vi "camera.vi"() -> (0 "color":string, 1 "result":bool, 2 "middle":T3(plugin-control))   [LabVIEW 2017]
panel:
  in  "range of detect screen":dbl=7.0
  in  "value of screen mid":dbl=160.0
  in  "distance between pole lines":sgl=2.0
  in  "Rectangle":T1={"Left"=150, "Top"=20, "Right"=170, "Bottom"=120, "Rotation"=0.0} {"Rotation" min=-90.0 max=90.0 step=1.0 format="%.2f"; "Left" scale=0.0..1024.0; "Right" scale=0.0..1024.0}
  out "inRange":bool
  out "not same":bool
  out "line_leftX":sgl
  out "line_rightX":sgl
  out "line_left":T2 {"Point2 (Real-World)"."Y" format="%.2f"; "Point2 (Real-World)"."X" format="%.2f"; "Point1 (Real-World)"."Y" format="%.2f"; "Point1 (Real-World)"."X" format="%.2f"; "Point2 (Pixels)"."Y" format="%.2f"; "Point2 (Pixels)"."X" format="%.2f"; "Point1 (Pixels)"."Y" format="%.2f"; "Point1 (Pixels)"."X" format="%.2f"}
  out "line_right":T2 {"Point2 (Real-World)"."Y" format="%.2f"; "Point2 (Real-World)"."X" format="%.2f"; "Point1 (Real-World)"."Y" format="%.2f"; "Point1 (Real-World)"."X" format="%.2f"; "Point2 (Pixels)"."Y" format="%.2f"; "Point2 (Pixels)"."X" format="%.2f"; "Point1 (Pixels)"."Y" format="%.2f"; "Point1 (Pixels)"."X" format="%.2f"}
  out "thresh":T3(plugin-control)
  in  "Stop (F)":bool
  out "Image Out":T3(plugin-control)
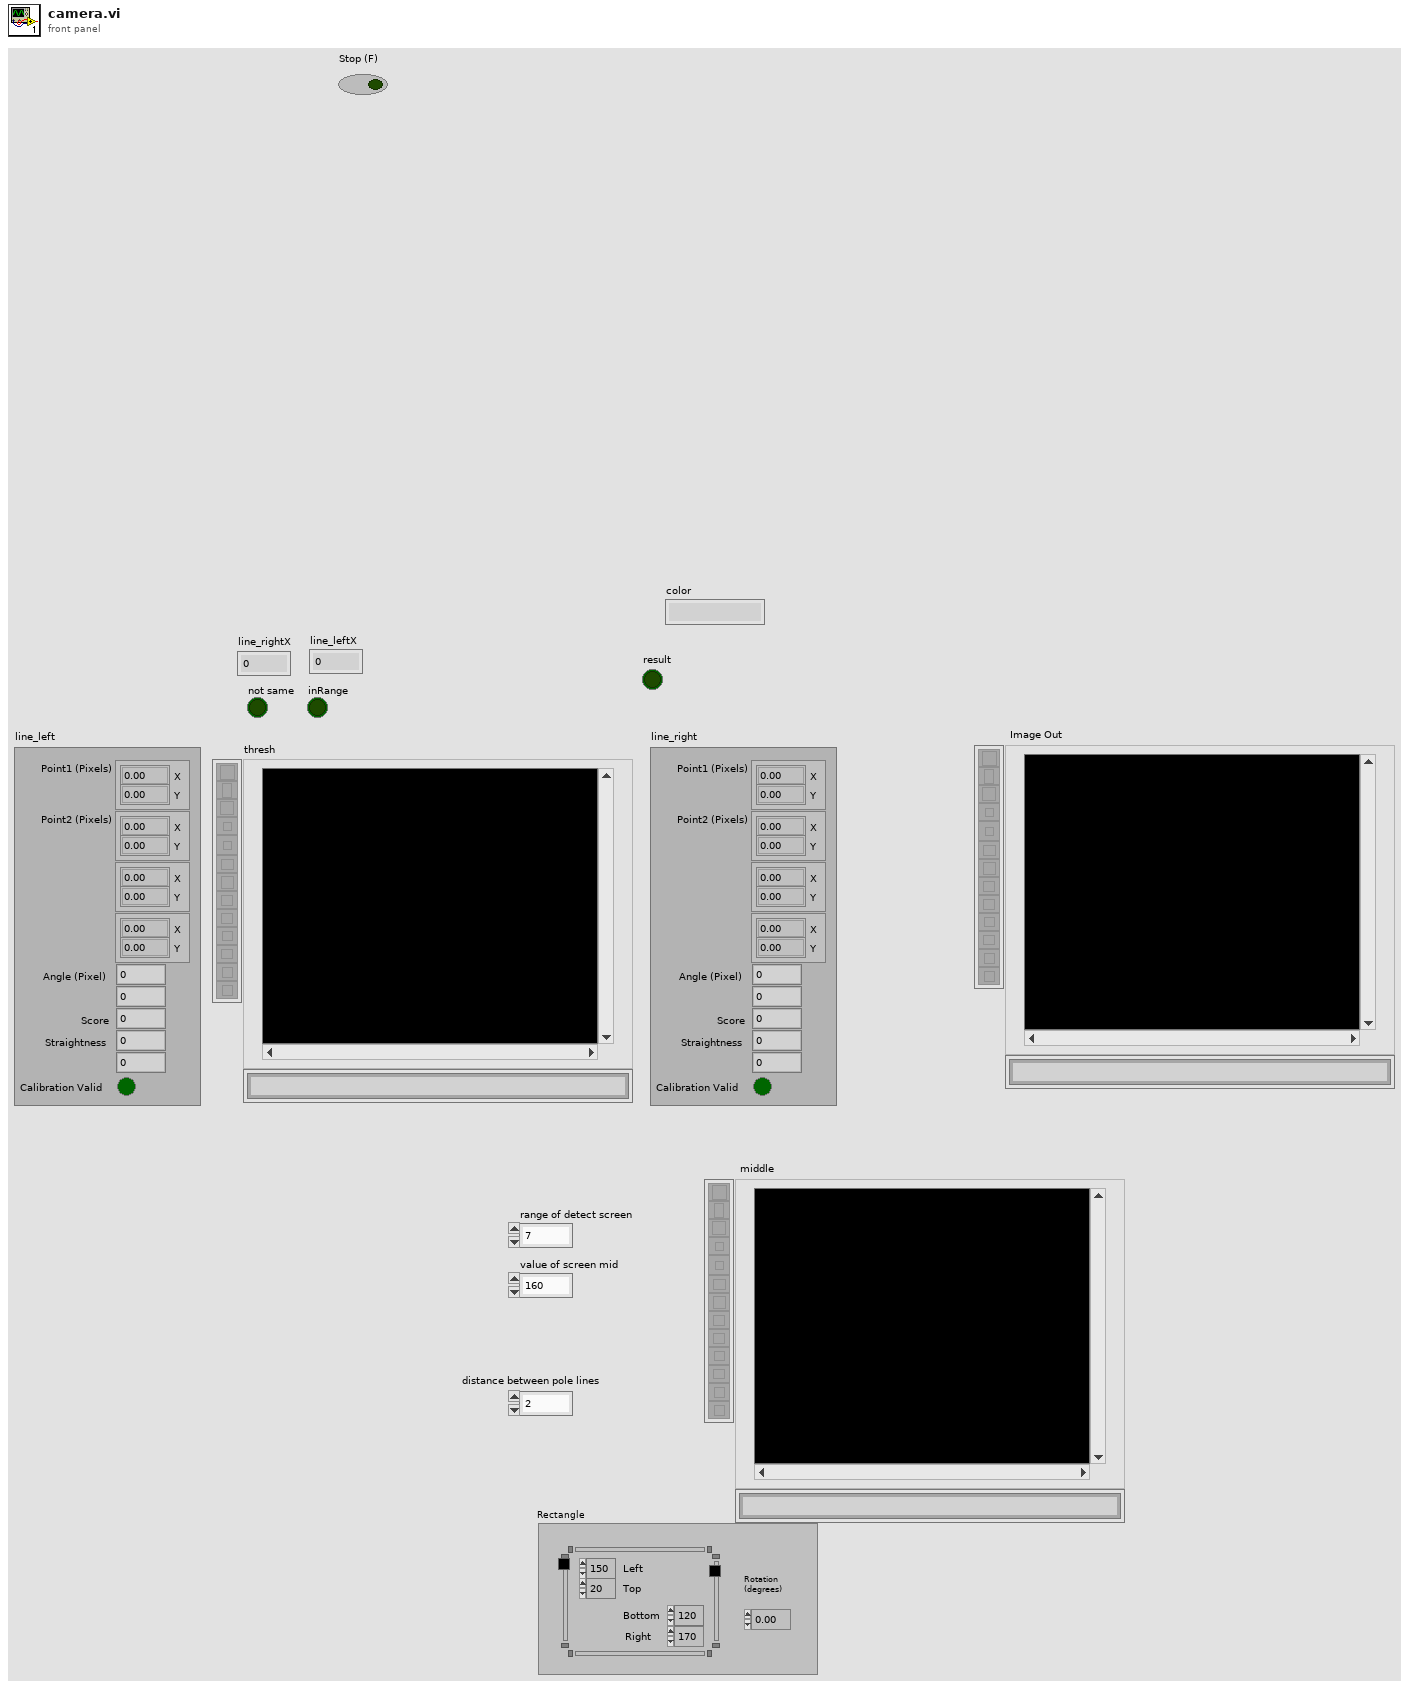
[diagram p1: front panel]
types:
  T1 = typedef "IMAQ Rectangle" = cluster{"Left":i32, "Top":i32, "Right":i32, "Bottom":i32, "Rotation":dbl}
  T2 = cluster{"Point1 (Pixels)":cluster{"X":sgl, "Y":sgl}, "Point2 (Pixels)":cluster{"X":sgl, "Y":sgl}, "Point1 (Real-World)":cluster{"X":sgl, "Y":sgl}, "Point2 (Real-World)":cluster{"X":sgl, "Y":sgl}, "Angle (Pixel)":dbl, "Angle (Real-World)":dbl, "Score":dbl, "Straightness":dbl, "Average SNR (db)":dbl, "Calibration Valid":bool}
  T3 = typedef "IMAQ Image.ctl" = refnum<image>
  T4 = typedef "Image Type" = u32
  T5 = typedef "ROI Descriptor" = cluster{"Global Rectangle":i32[], "Contours":cluster{"ID":enum32{"External", "Internal"}, "Type":u32, "Coordinates":i32[]}[]}
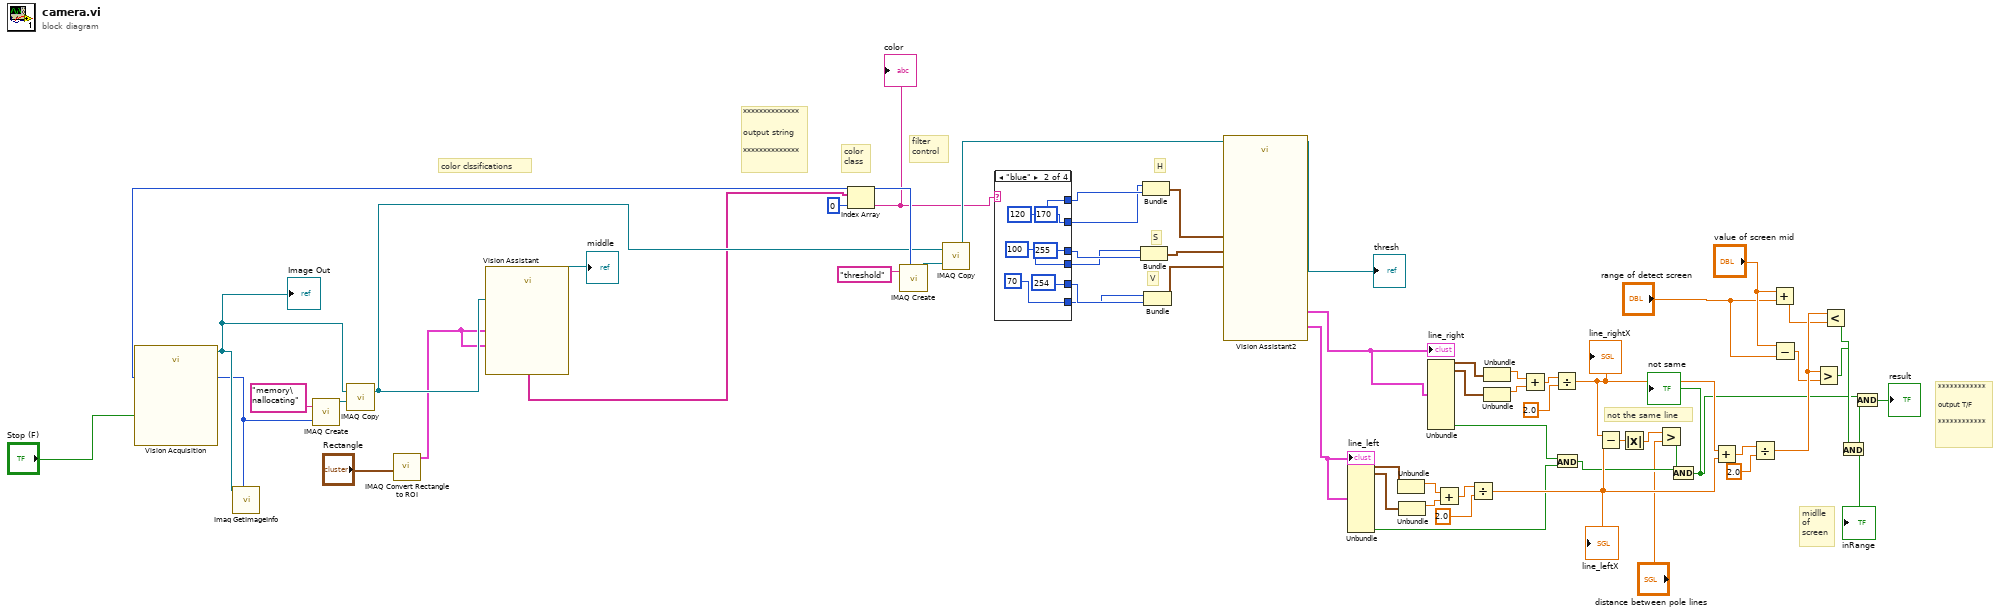
[diagram p0: block diagram]
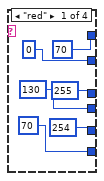
[diagram p2: hidden frame]
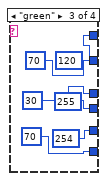
[diagram p3: hidden frame]
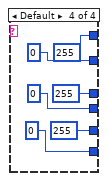
[diagram p4: hidden frame]
diagram:
  # "**************\n\noutput string\n\n**************"
  # "************\n\noutput T/F\n\n************"
  # "color clssifications"
  # "midlle\nof\nscreen"
  # "not the same line"
  # "filter\ncontrol"
  # "color\nclass"
  # "V"
  # "S"
  # "H"
  n1 = call "Vision Acquisition"("Stop (F)"="Stop (F)") -> ("Image Out"=w57:T3)  [unwired: 24 in, 2 out]
  "Image Out" <- w57
  n2 = call "Imaq GetImageInfo"("Image"=w57) -> ("Image Type"=w40:T4)  [unwired: 3 in, 7 out]
  n3 = call "IMAQ Create"("Image Name"="memory\nallocating", "Image Type"=w40) -> ("New Image"=w59:T3)  [unwired: 3 in, 1 out]
  n4 = call "IMAQ Copy"("Image Dst"=w59, "Image Src"=w57) -> ("Image Dst Out"=w39:T3)  [unwired: 4 in, 1 out]
  n5 = call "IMAQ Convert Rectangle to ROI"("Rectangle"="Rectangle") -> ("ROI Descriptor"=w7:T5)  [unwired: 8 in, 1 out]
  n6 = call "Vision Assistant"("Image In"=w39, "ROI Descriptor (Color Classification 1)"=w7, "ROI Descriptor (Image Mask 1)"=w7) -> ("Image Out"=→"middle":T3, "Classes (Color Classification 1)"=w9:string[])  [unwired: 22 in, 1 out]
  n7 = Index Array(array=w9, index=0) -> (element=w8:string)
  "color" <- w8
  n8 = call "IMAQ Create"("Image Name"="threshold", "Image Type"=w40) -> ("New Image"=w55:T3)  [unwired: 3 in, 1 out]
  n9 = call "IMAQ Copy"("Image Dst"=w55, "Image Src"=w39) -> ("Image Dst Out"=w51:T3)  [unwired: 4 in, 1 out]
  n10 = case shown="\"blue\"" w8 {
    tunnel: [0 120 70 0] -> w45
    tunnel: [70 170 120 255] -> w46
    tunnel: [130 100 30 0] -> w43
    tunnel: [255 255 255 255] -> w44
    tunnel: [70 70 70 0] -> w41
    tunnel: [254 254 254 255] -> w42
    frame "red" {
    }
    frame "blue" {
    }
    frame "green" {
    }
    frame Default {
    }
  }
  n11 = Bundle(w43, w44) -> (w48:cluster{i32, i32})  [unwired: 1 in]
  n12 = Bundle(w45, w46) -> (w49:cluster{i32, i32})  [unwired: 1 in]
  n13 = Bundle(w41, w42) -> (w47:cluster{i32, i32})  [unwired: 1 in]
  n14 = call "Vision Assistant2"("Image In"=w51, "Red or Hue Range (Color Threshold 1)"=w49, "Green or Sat Range (Color Threshold 1)"=w48, "Blue or Luma or Val or Inten Range (Color Threshold 1)"=w47) -> ("Image Out"=→"thresh":T3, "Straight Edge (Find Straight Edge 1)"=w50:T2, "Straight Edge (Copy of Find Straight Edge 1)"=w38:T2)  [unwired: 20 in, 1 out]
  "line_right" <- w50
  "line_left" <- w38
  n15 = Unbundle(w38) -> ("Point1 (Pixels)"=w36:cluster{"X":sgl, "Y":sgl}, "Point2 (Pixels)"=w35:cluster{"X":sgl, "Y":sgl}, "Calibration Valid"=w15:bool)  [unwired: 7 out]
  n16 = Unbundle(w36) -> ("X"=w34:sgl)  [unwired: 1 out]
  n17 = Unbundle(w35) -> ("X"=w33:sgl)  [unwired: 1 out]
  n18 = Unbundle(w50) -> ("Point1 (Pixels)"=w52:cluster{"X":sgl, "Y":sgl}, "Point2 (Pixels)"=w37:cluster{"X":sgl, "Y":sgl}, "Calibration Valid"=w16:bool)  [unwired: 7 out]
  n19 = Add(x=w34, y=w33) -> (x+y=w32:sgl)
  n20 = Divide(x=w32, y=sgl 2.0) -> (x/y=w20:sgl)
  "line_leftX" <- w20
  n21 = Unbundle(w52) -> ("X"=w28:sgl)  [unwired: 1 out]
  n22 = Unbundle(w37) -> ("X"=w27:sgl)  [unwired: 1 out]
  n23 = Add(x=w28, y=w27) -> (x+y=w30:sgl)
  n24 = Divide(x=w30, y=sgl 2.0) -> (x/y=w21:sgl)
  "line_rightX" <- w21
  n25 = And(x=w16, y=w15) -> (x .and. y?=w14:bool)
  n26 = Subtract(x=w21, y=w20) -> (x-y=w19:sgl)
  n27 = Absolute Value(x=w19) -> (abs(x)=w17:sgl)
  n28 = Greater?(x=w17, y="distance between pole lines") -> (0:w13:bool)
  n29 = And(x=w14, y=w13) -> (x .and. y?=w12:bool)
  "not same" <- w12
  n30 = Add(x=w21, y=w20) -> (x+y=w26:sgl)
  n31 = Divide(x=w26, y=sgl 2.0) -> (x/y=w24:sgl)
  n32 = Add(x="value of screen mid", y="range of detect screen") -> (x+y=w3:dbl)
  n33 = Subtract(x="value of screen mid", y="range of detect screen") -> (x-y=w4:dbl)
  n34 = Greater?(x=w24, y=w4) -> (0:w22:bool)
  n35 = Less?(x=w24, y=w3) -> (x < y?=w23:bool)
  n36 = And(x=w23, y=w22) -> (x .and. y?=w18:bool)
  "inRange" <- w18
  n37 = And(x=w12, y=w18) -> (x .and. y?=→"result":bool)
